vi "PCI1220U使能.vi"(10 "使能":bool, 11 "AxisHandle IN":u32) -> (3 "AxisHandle OUT":u32)   [LabVIEW 2013]
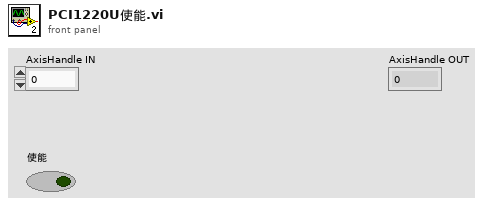
[diagram p1: front panel]
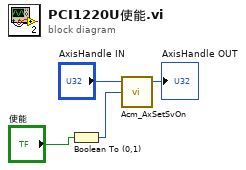
[diagram p0: block diagram]
diagram:
  n1 = Boolean To (0,1)(Boolean="使能") -> (0, 1=w1:i16)
  n2 = call <userlib>:"Acm_AxSetSvOn.vi"("OnOff"=w1, "AxisHandle"="AxisHandle IN") -> ("AxisHandle"=→"AxisHandle OUT":u32)  [unwired: 1 in, 2 out]
